vi "Read Gyro Range.vi"(8 "error in (no error)":errorcluster, 11 "LSM9DS1 IMU in":refnum<class "LSM9DS1 IMU.lvclass">) -> (0 "error out":errorcluster, 2 "Gyro Range":T1, 3 "LSM9DS1 IMU out":refnum<class "LSM9DS1 IMU.lvclass">)   [LabVIEW 2020, in "LSM9DS1 IMU.lvclass"]
uses:
  LSM9DS1 IMU.lvclass
  Gyro Range.ctl
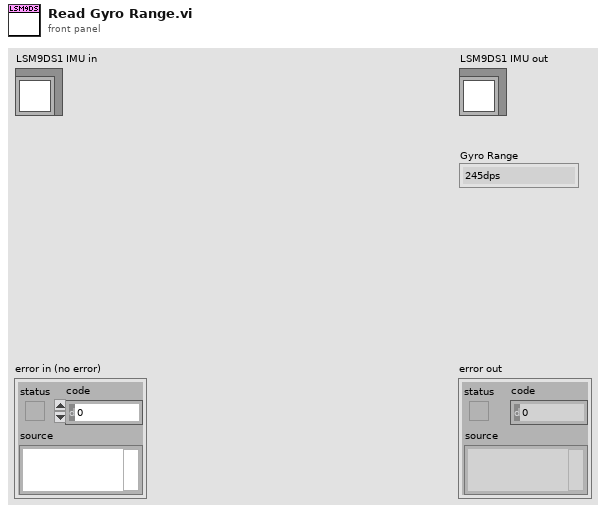
[diagram p1: front panel]
types:
  T1 = typedef "LSM9DS1 IMU.lvclass/Gyro Range.ctl" = enum16{"245dps", "500dps", "2000dps"}
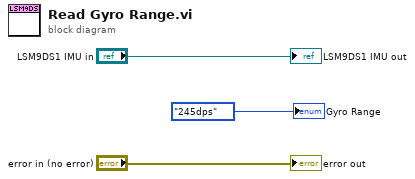
[diagram p0: block diagram]
diagram:
  "error out" <- "error in (no error)"
  "LSM9DS1 IMU out" <- "LSM9DS1 IMU in"
  "Gyro Range" <- Gyro_Range."245dps" ("Gyro Range")
